vi "Transform2d_Plus.vi"(9 "otherTRANSFORM":T1={"TRANSLATION"={"X"=0.0, "Y"=0.0}, "ROTATION"={"VALUE"=0.0, "COS"=1.0, "SIN"=0.0}} {"ROTATION"."SIN" format="%13.4f"; "ROTATION"."COS" format="%13.4f"; "ROTATION"."VALUE" format="%13.4f"; "TRANSLATION"."Y" format="%14.3f"; "TRANSLATION"."X" format="%14.3f"}, 11 "inTRANSFORM":T1={"TRANSLATION"={"X"=0.0, "Y"=0.0}, "ROTATION"={"VALUE"=0.0, "COS"=1.0, "SIN"=0.0}} {"ROTATION"."SIN" format="%13.4f"; "ROTATION"."COS" format="%13.4f"; "ROTATION"."VALUE" format="%13.4f"; "TRANSLATION"."Y" format="%14.3f"; "TRANSLATION"."X" format="%14.3f"}) -> (3 "TRANSFORM":T1 {"ROTATION"."SIN" format="%13.4f"; "ROTATION"."COS" format="%13.4f"; "ROTATION"."VALUE" format="%13.4f"; "TRANSLATION"."Y" format="%14.3f"; "TRANSLATION"."X" format="%14.3f"})   [LabVIEW 2019, in "Trajectory_Library.lvlib"]
doc: "Composes two transformations.\n\nParameters:\n - IN TRANSFORM - This TRANSFORM data structure\n - other Transform -- The transform to compose with this one.\n\nResults:\n - OUT TRANSFORM - The composition of the two transformations."
uses:
  Trajectory_Library.lvlib
  TRANSFORM2D.ctl
  TRANSLATION2D.ctl
  ROTATION2D.ctl
  Rotation2d_UnaryMinus.vi
  Translation2d_RotateBy.vi
  Translation2d_Minus.vi
  Rotation2d_Minus.vi
  Rotation2d_CreateAngle.vi
  Translation2d_Create.vi
  Translation2d_Plus.vi
  Rotation2d_Plus.vi
  Pose2d_New_TRRO.vi
  Rotation2d_RotateBy.vi
  Rotation2d_CreateXY.vi
  Util_CalcDist.vi
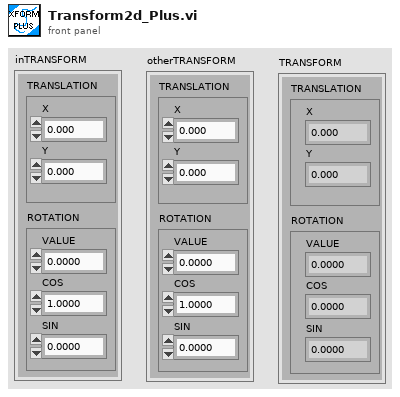
[diagram p1: front panel]
types:
  T1 = typedef "Trajectory_Library.lvlib/TRANSFORM2D.ctl" = cluster{"TRANSLATION":T2, "ROTATION":T3}
  T2 = typedef "Trajectory_Library.lvlib/TRANSLATION2D.ctl" = cluster{"X":dbl, "Y":dbl}
  T3 = typedef "Trajectory_Library.lvlib/ROTATION2D.ctl" = cluster{"VALUE":dbl, "COS":dbl, "SIN":dbl}
  T4 = typedef "Trajectory_Library.lvlib/POSE2D.ctl" = cluster{"TRANSLATION":T2, "ROTATION":T3}
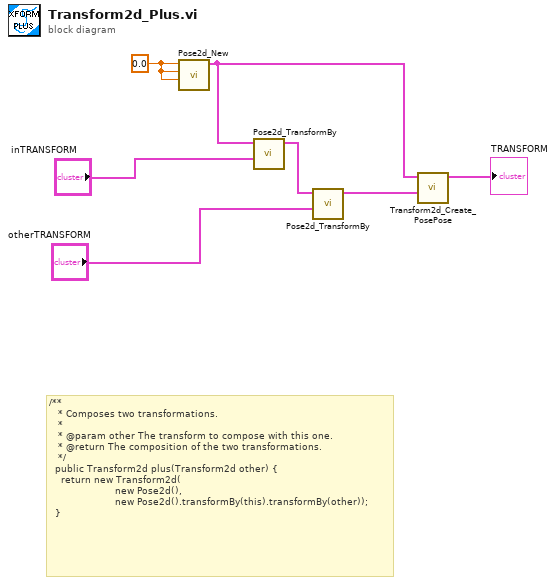
[diagram p0: block diagram]
diagram:
  w7 = 0.0 ("X")
  # "/**\n   * Composes two transformations.\n   *\n   * @param other The transform to compose with this one.\n   * @return The composition of the two transformations.\n   */\n  public Transform2d plus(Transform2d other) {\n    return new Transform2d(\n                      new Pose2d(), \n                      new Pose2d().transformBy(this).transformBy(other));\n  }"
  n1 = call "Pose2d_New.vi"("Heading"=w7, "Y"=w7, "X"=w7) -> ("out POSe"=w6:T4)  [unwired: 8 in]
  n2 = call "Pose2d_TransformBy.vi"("other TRANSFORM"="inTRANSFORM", "in POSE"=w6) -> ("out POSE"=w5:T4)  [unwired: 9 in]
  n3 = call "Pose2d_TransformBy.vi"("other TRANSFORM"="otherTRANSFORM", "in POSE"=w5) -> ("out POSE"=w4:T4)  [unwired: 9 in]
  n4 = call "Transform2d_Create_PosePose.vi"("last POSE"=w4, "initial POSE"=w6) -> ("TRANSFORM"=→"TRANSFORM":T1)  [unwired: 9 in]
